vi "sub_error_data-conversion.vi"(10 "name":string, 11 "error status":bool) -> (2 "check result string":string, 3 "error conversion out":u16(ring))   [LabVIEW 2019]
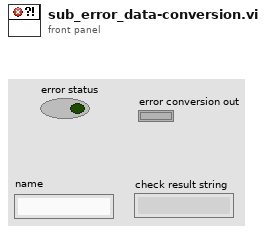
[diagram p1: front panel]
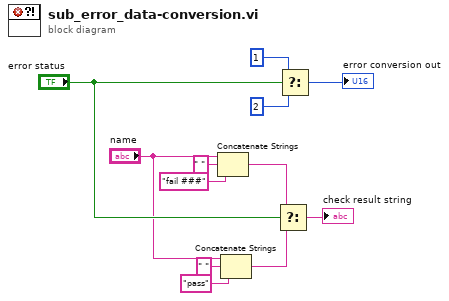
[diagram p0: block diagram]
diagram:
  n1 = Concatenate Strings("name", " " ("string"), "fail ###" ("string")) -> (w6:string)
  n2 = Concatenate Strings("name", " " ("string"), "pass" ("string")) -> (w2:string)
  n3 = Select(t=w6, s="error status", f=w2) -> (s? t:f=→"check result string":string)
  n4 = Select(t=u16 1 ("VLP16"), s="error status", f=u16 2 ("VLP16")) -> (s? t:f=→"error conversion out":u16)
